vi "IOSetTool.vi"() -> ()   [LabVIEW 2021]
doc: "Use this template to build a producer/consumer design pattern with events to produce queue items. Use this design pattern instead of the User Interface Event Handler pattern for user interfaces when you want to execute code asynchronously in response to an event without slowing the user interface responsiveness."
panel:
  in  "Select JSON File":bool
  out "Function String":string
  in  "Export":bool
  in  "Funtion Type":enum32{"type1", "type2"}(radio)
  in  "Reinitialize Values to Default":bool
  in  "Deselect All":bool
  in  "Select All":bool
  in  "IO_Set":i32[](listbox)
  # "1.Run the VI.\n2.Select IOs.JSON file.\n3.Select variants and set value.\n4.Select function type.\n5.Click the 'Export' button and get the function string.\n\nTips:\nFor the bit type, 0 is false and other numbers is true."
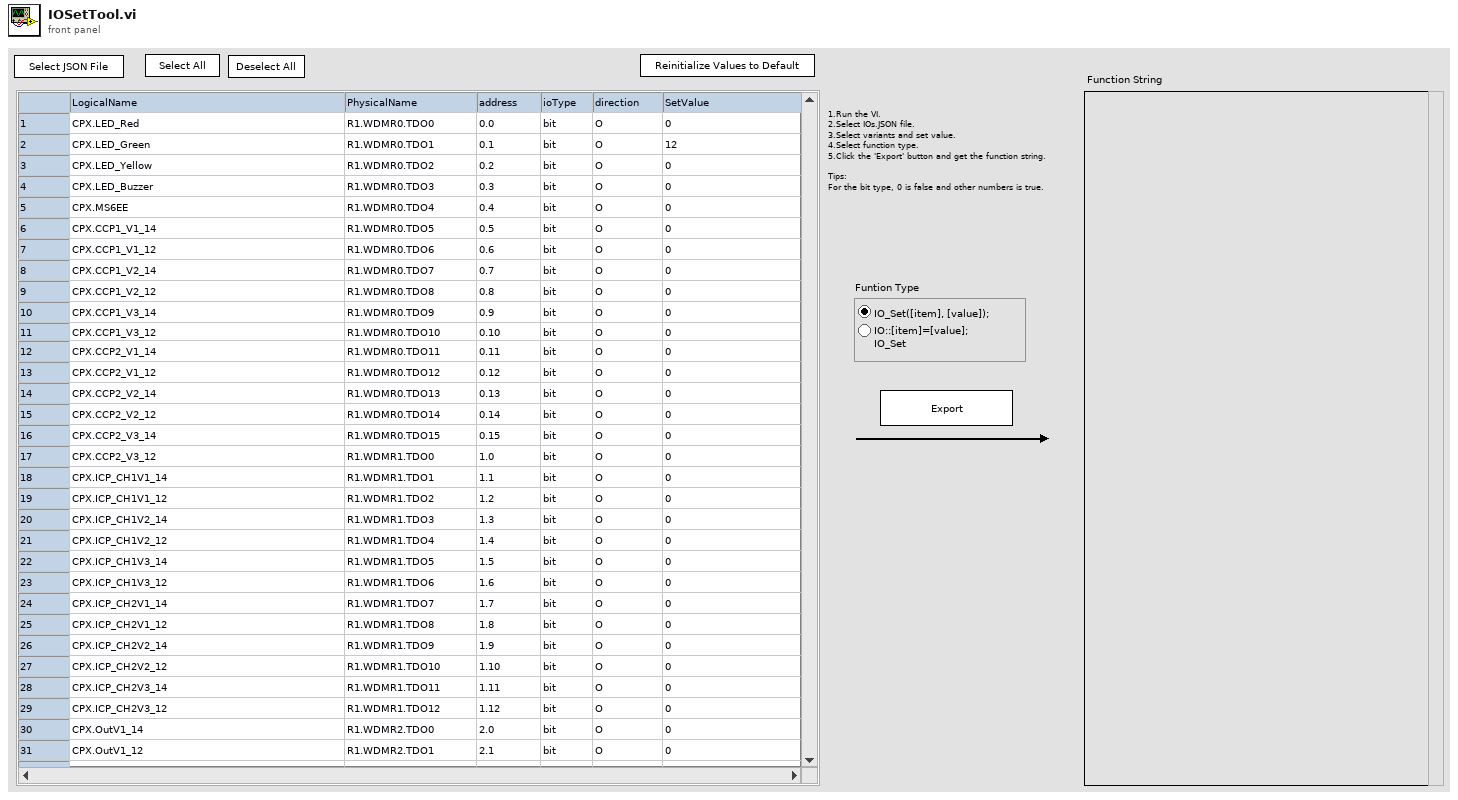
[diagram p1: front panel]
types:
  T1 = enum8{"Enabled", "Disabled", "Disabled and Grayed Out"}
  T2 = cluster{"items":cluster{"LogicalName":string, "PhysicalName":string, "address":string, "ioType":string, "direction":string}[]}
  T3 = enum16{"open", "replace", "create", "open or create", "replace or create", "replace or create with confirmation"}
  T4 = typedef "LVPoint32TypeDef.ctl" = cluster{"Horizontal":i32, "Vertical":i32}
  T5 = typedef "LVRowAndColumnTypeDef.ctl" = cluster{"Row":i32, "Column":i32}
  T6 = cluster{"LogicalName":string, "PhysicalName":string, "address":string, "ioType":string, "direction":string}[]
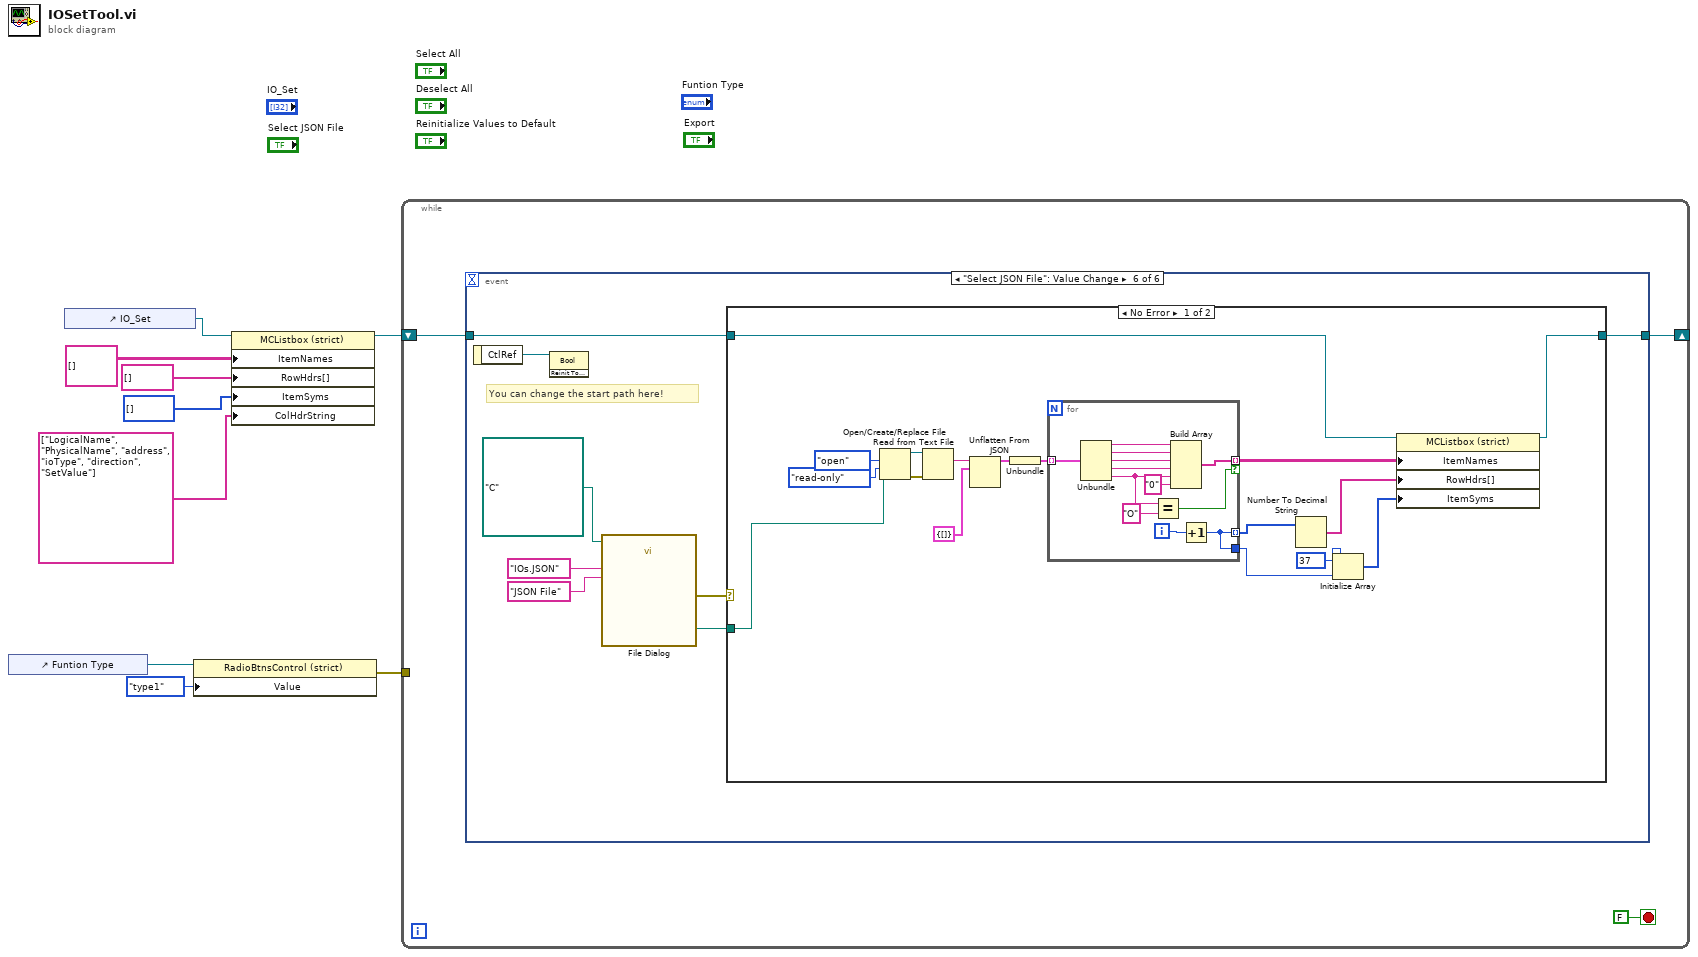
[diagram p0: block diagram]
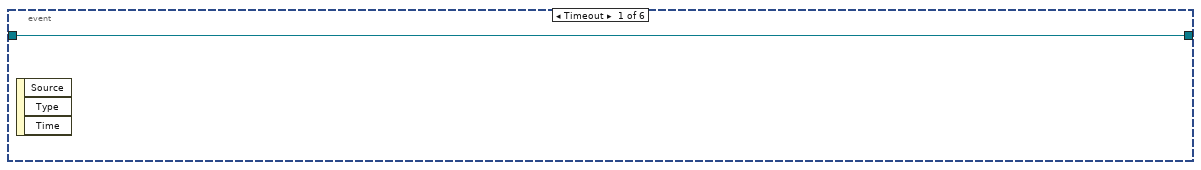
[diagram p2: hidden frame]
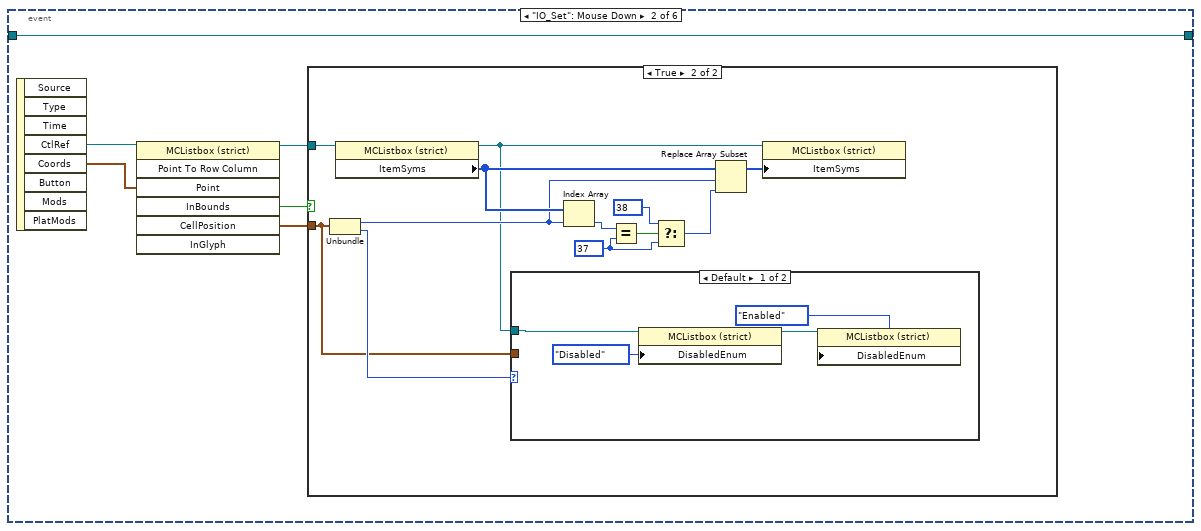
[diagram p3: hidden frame]
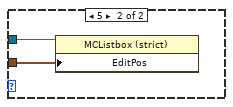
[diagram p5: hidden frame]
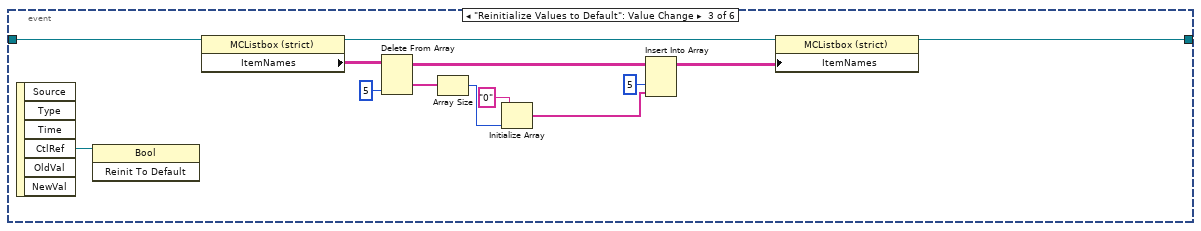
[diagram p6: hidden frame]
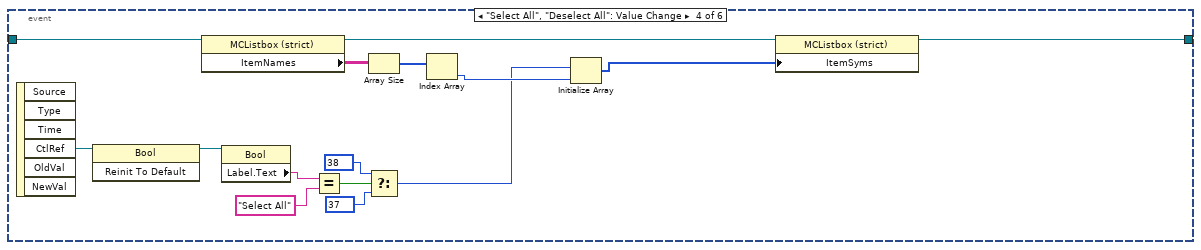
[diagram p7: hidden frame]
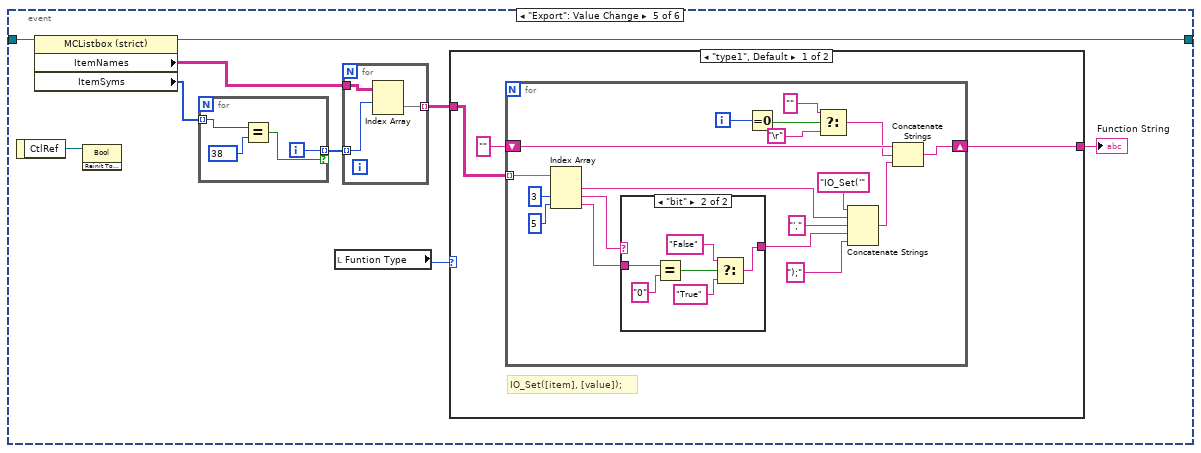
[diagram p8: hidden frame]
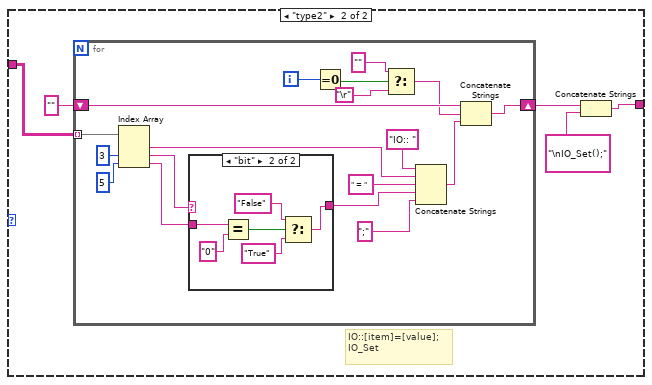
[diagram p10: hidden frame]
diagram:
  n1 = control-ref of="Funtion Type"() -> (w9:refnum<vi>)
  n2 = control-ref of="IO_Set"() -> (w3:refnum<vi>)
  n3 = property class="RadioBtnsControl (strict)"(reference=w9, "Value"=enum32{"type1", "type2"}."type1") -> (error out=w7:errorcluster)  [unwired: 1 in, 1 out]
  n4 = property class="MCListbox (strict)"(reference=w3, "ItemNames"=string[][] [] ("Item Names"), "RowHdrs[]"=string[] [] ("Row Header Strings[]"), "ItemSyms"=i32[] [] ("Item Symbols"), "ColHdrString"=string[] ["LogicalName", "PhysicalName", "address", "ioType", "direction", "SetValue"] ("Column Header Strings[]")) -> (reference out=w2:refnum<vi>)  [unwired: 1 in, 1 out]
  n5 = while {
    shift-right: [w10] -> _
    shift-left: w2 -> [w11]
    tunnel: w7 -> [_]
    stop <- FALSE stop-if-true
    n6 = event shown="[5] \"Select JSON File\": Value Change" {
      selector: _ -> [_ _ _ _ _ _]
      dyn-events: _ -> [_ _ _ _ _ _]
      timeout: _ -> [_ _ _ _ _ _]
      tunnel: w11 -> [w13 w14 w49 w64 w73 w141]
      tunnel: [w13 w14 w47 w62 w69 w140] -> w10
      event Timeout {
        n7 = event-data() -> ()  [unwired: 1 in, 3 out]
      }
      event "IO_Set": Mouse Down {
        n8 = event-data() -> ("CtlRef"=w19:refnum<vi>, "Coords"=w18:T4)  [unwired: 1 in, 6 out]
        n9 = invoke class="MCListbox (strict)" method="Point To Row Column"(reference=w19, "Point"=w18) -> (reference out=w15:refnum<vi>, "InBounds"=w17:bool, "CellPosition"=w16:T5)  [unwired: 5 in, 4 out]
        n10 = case shown="True" w17 {
          tunnel: w16 -> [_ w20]
          tunnel: w15 -> [_ w31]
          frame False {
          }
          frame True {
            w27 = 37
            n11 = Unbundle(w20) -> ("Row"=w24:i32, "Column"=w22:i32)
            n12 = property class="MCListbox (strict)"(reference=w31) -> (reference out=w21:refnum<vi>, "ItemSyms"=w26:i32[])  [unwired: 1 in, 1 out]
            n13 = case shown="Default" w22 {
              tunnel: w21 -> [w35 w37]
              tunnel: w20 -> [_ w36]
              frame Default {
                n14 = property class="MCListbox (strict)"(reference=w35, "DisabledEnum"=T1."Disabled" ("Disabled")) -> (reference out=w33:refnum<vi>)  [unwired: 1 in, 1 out]
                n15 = property class="MCListbox (strict)"(reference=w33, "DisabledEnum"=T1."Enabled" ("Disabled")) -> ()  [unwired: 1 in, 2 out]
              }
              frame 5 {
                n16 = property class="MCListbox (strict)"(reference=w37, "EditPos"=w36) -> ()  [unwired: 1 in, 2 out]
              }
            }
            n17 = Index Array(array=w26, index=w24) -> (element=w30:i32)
            n18 = Equal?(x=w30, y=w27) -> (x = y?=w29:bool)
            n19 = Select(t=38, s=w29, f=w27) -> (s? t:f=w25:i32)
            n20 = Replace Array Subset(array=w26, new element=w25, index=w24) -> (w23:i32[])
            n21 = property class="MCListbox (strict)"(reference=w21, "ItemSyms"=w23) -> ()  [unwired: 1 in, 2 out]
          }
        }
      }
      event "Reinitialize Values to Default": Value Change {
        n22 = event-data() -> ("CtlRef"=w50:refnum<vi>)  [unwired: 1 in, 5 out]
        n23 = invoke class="Bool" method="Reinit To Default"(reference=w50) -> ()  [unwired: 2 in, 3 out]
        n24 = property class="MCListbox (strict)"(reference=w49) -> (reference out=w48:refnum<vi>, "ItemNames"=w46:string[][])  [unwired: 1 in, 1 out]
        n25 = Delete From Array(array=w46, index (col)=5 ("disabled index (col)")) -> (deleted portion=w43:string[], array with subset deleted=w44:string[][])  [unwired: 2 in]
        n26 = Array Size(array=w43) -> (size(s)=w42:i32)
        n27 = Initialize Array("0", w42) -> (w40:string[])
        n28 = Insert Into Array(array=w44, index (col)=5 ("disabled index (col)"), new element=w40) -> (w38:string[][])  [unwired: 1 in]
        n29 = property class="MCListbox (strict)"(reference=w48, "ItemNames"=w38) -> (reference out=w47:refnum<vi>)  [unwired: 1 in, 1 out]
      }
      event "Select All", "Deselect All": Value Change {
        n30 = event-data() -> ("CtlRef"=w65:refnum<vi>)  [unwired: 1 in, 5 out]
        n31 = invoke class="Bool" method="Reinit To Default"(reference=w65) -> (reference out=w59:refnum<vi>)  [unwired: 2 in, 2 out]
        n32 = property class="MCListbox (strict)"(reference=w64) -> (reference out=w63:refnum<vi>, "ItemNames"=w61:string[][])  [unwired: 1 in, 1 out]
        n33 = property class="Bool"(reference=w59) -> ("Label.Text"=w58:string)  [unwired: 1 in, 2 out]
        n34 = Equal?(x=w58, y="Select All") -> (x = y?=w56:bool)
        n35 = Array Size(array=w61) -> (size(s)=w60:i32[])
        n36 = Select(t=38, s=w56, f=37) -> (s? t:f=w52:i32)
        n37 = Index Array(array=w60) -> (element=w53:i32)  [unwired: 1 in]
        n38 = Initialize Array(w52, w53) -> (w51:i32[])
        n39 = property class="MCListbox (strict)"(reference=w63, "ItemSyms"=w51) -> (reference out=w62:refnum<vi>)  [unwired: 1 in, 1 out]
      }
      event "Export": Value Change {
        n40 = event-data() -> ("CtlRef"=w74:refnum<vi>)  [unwired: 1 in]
        n41 = property class="MCListbox (strict)"(reference=w73) -> (reference out=w69:refnum<vi>, "ItemNames"=w70:string[][], "ItemSyms"=w72:i32[])  [unwired: 1 in, 1 out]
        n42 = invoke class="Bool" method="Reinit To Default"(reference=w74) -> ()  [unwired: 2 in, 3 out]
        n43 = for {
          tunnel: w72 -> [w139] mode=indexing
          tunnel: [w137] -> w71 mode=indexing if=w136
          i -> [w137]
          n44 = Equal?(x=w139, y=38) -> (x = y?=w136:bool)
        }
        n45 = local read "Funtion Type"() -> (w68:enum32{"type1", "type2"})
        n46 = for {
          tunnel: w71 -> [w134] mode=indexing
          tunnel: w70 -> [w135]
          tunnel: [w133] -> w67 mode=indexing
          n47 = Index Array(array=w135, index (row)=w134) -> (element=w133:string[])  [unwired: 1 in]
        }
        n48 = case shown="\"type1\", Default" w68 {
          tunnel: w67 -> [w77 w106]
          tunnel: [w75 w104] -> w66
          frame "type1", Default {
            # "IO_Set([item], [value]);"
            n49 = for {
              tunnel: w77 -> [w92] mode=indexing
              shift-right: [w80] -> w75
              shift-left: "" ("element") -> [w81]
              i -> [w85]
              n50 = Index Array(array=w92, index #2=3 ("index"), index #3=5 ("index")) -> (element #1=w91:string, element #2=w89:string, element #3=w86:string)  [unwired: 1 in]
              n51 = case shown="\"bit\"" w89 {
                tunnel: [w96 w97] -> w88
                tunnel: w86 -> [w96 w102]
                frame Default {
                }
                frame "bit" {
                  n52 = Equal?(x=w102, y="0") -> (x = y?=w100:bool)
                  n53 = Select(t="False" ("y"), s=w100, f="True") -> (s? t:f=w97:string)
                }
              }
              n54 = Equal To 0?(x=w85) -> (x = 0?=w84:bool)
              n55 = Select(t="" ("string"), s=w84, f="\r") -> (s? t:f=w78:string)
              n56 = Concatenate Strings("IO_Set('" ("string"), w91, "'," ("string"), w88, ");" ("string")) -> (w79:string)
              n57 = Concatenate Strings(w81, w78, w79) -> (w80:string)
            }
          }
          frame "type2" {
            # "IO::[item]=[value];\nIO_Set"
            n58 = for {
              tunnel: w106 -> [w122] mode=indexing
              shift-right: [w110] -> w105
              shift-left: "" ("element") -> [w111]
              i -> [w115]
              n59 = Index Array(array=w122, index #2=3 ("index"), index #3=5 ("index")) -> (element #1=w121:string, element #2=w119:string, element #3=w116:string)  [unwired: 1 in]
              n60 = case shown="\"bit\"" w119 {
                tunnel: [w126 w127] -> w118
                tunnel: w116 -> [w126 w132]
                frame Default {
                }
                frame "bit" {
                  n61 = Equal?(x=w132, y="0") -> (x = y?=w130:bool)
                  n62 = Select(t="False" ("y"), s=w130, f="True") -> (s? t:f=w127:string)
                }
              }
              n63 = Equal To 0?(x=w115) -> (x = 0?=w114:bool)
              n64 = Select(t="" ("string"), s=w114, f="\r") -> (s? t:f=w108:string)
              n65 = Concatenate Strings("IO:: " ("string"), w121, " = " ("string"), w118, ";" ("string")) -> (w109:string)
              n66 = Concatenate Strings(w111, w108, w109) -> (w110:string)
            }
            n67 = Concatenate Strings(w105, "\nIO_Set();" ("string")) -> (w104:string)
          }
        }
        "Function String" <- w66
      }
      event "Select JSON File": Value Change {
        # "You can change the start path here!"
        n68 = event-data() -> ("CtlRef"=w147:refnum<vi>)  [unwired: 1 in]
        n69 = invoke class="Bool" method="Reinit To Default"(reference=w147) -> ()  [unwired: 2 in, 3 out]
        n70 = call "File Dialog"("start path"=path "C:/", "pattern (all files)"="IOs.JSON", "pattern label"="JSON File") -> ("selected path"=w142:path, "error out"=w143:errorcluster)  [unwired: 9 in, 2 out]
        n71 = case shown="No Error" w143 {
          tunnel: w142 -> [w150 _]
          tunnel: w141 -> [w149 w177]
          tunnel: [w148 w177] -> w140
          frame No Error {
            n72 = Open/Create/Replace File(file path (use dialog)=w150, operation (0:open)=T3."open", access (0:read/write)=enum16{"read/write", "read-only", "write-only"}."read-only") -> (refnum out=w155:refnum<file>, error out=w156:errorcluster)  [unwired: 3 in, 1 out]
            n73 = Read from Text File(file (use dialog)=w155, error in=w156) -> (text=w157:string)  [unwired: 2 in, 3 out]
            n74 = Unflatten From JSON(JSON string=w157, type and defaults=T2 {"items"=[]} ("json")) -> (value=w158:T2)  [unwired: 5 in, 1 out]
            n75 = Unbundle(w158) -> ("items"=w159:T6)
            n76 = for {
              tunnel: w159 -> [w176] mode=indexing
              tunnel: [w171] -> w160 mode=indexing if=w166
              tunnel: [w169] -> w161 mode=indexing
              tunnel: [w169] -> w163
              i -> [w170]
              n77 = Unbundle(w176) -> ("LogicalName"=w175:string, "PhysicalName"=w174:string, "address"=w173:string, "ioType"=w172:string, "direction"=w168:string)
              n78 = Equal?(x=w168, y="O") -> (x = y?=w166:bool)
              n79 = Build Array(w175, w174, w173, w172, w168, "0" ("element")) -> (w171:string[])
              n80 = Increment(x=w170) -> (x+1=w169:i32)
            }
            n81 = Number To Decimal String(number=w161) -> (decimal integer string=w162:string[])  [unwired: 1 in]
            n82 = Initialize Array(37, w163) -> (w164:i32[])
            n83 = property class="MCListbox (strict)"(reference=w149, "ItemNames"=w160, "RowHdrs[]"=w162, "ItemSyms"=w164) -> (reference out=w148:refnum<vi>)  [unwired: 1 in, 1 out]
          }
          frame Error {
          }
        }
      }
    }
  }
